vi "TekAFG3102_2.vi"() -> ()   [LabVIEW 2015]
uses:
  Shared program Control/loop state machine.ctl
  NetworkStream/NetworkStreamReceiverState.ctl
  NetworkStream/NetworkStreamStateMachineVariable.ctl
  NetworkStream/NetworkStreamData.ctl
  Shared program Control/MasterStatus.ctl
  <vilib>/dex/Stream Element Allocation Mode.ctl
  ICcamera/MyToolsFunction.lvlib
  Tek shared libraries/ArbitraryFunctions.lvlib
  NetworkStream/NetworkStream.lvlib
  Shared program Control/MySharedVariables.lvlib
  Tek shared libraries/SerialCommunication.lvlib
panel:
  out "error out 2":errorcluster caption="error out" {"code" format="%.0x"}
  in  "get tek parameters":bool
  out "error out":errorcluster {"code" format="%.0x"}
  in  "visa":bool
  out "Read Buffer":string
  in  "Write Buffer (\"\")":string="*IDN?"
  out "sequence number":u64
  in  "user waveform":bool
  in  "Channel 1 ON/OFF":bool
  in  "resource name":refnum<k15>
  in  "Stop Button":bool
  out "Session Hash":u64
  out "Network Stream State Indicator":T1
  in  "slot to load (update first)":i32(ring) items=["Slot 1", "Slot 2", "Slot 3", "Slot 4"]
  in  "channels":enum32{"active channel", ""}(radio)
  in  "Tab Control":T2(tab)
  in  "CM cluster":T3={"Frequency (Hz)"=80000000.0, "Amplitude (V)"=0.2, "Phase (°)"=0.0, "Offset (Volt)"=0.0, "Standard waveform (1: Sine)"=1, "output mode"=0, "Modulation Waveform (1: Sine)"=1} {"Modulation Waveform (1: Sine)" items=["Sine"=1, "Square"=2, "Triangle"=3, "Ramp Up"=4, "Ramp Down"=5, "Noise"=100, "Arbitrary User1"=200, "Arbitrary User2"=201, "Arbitrary User3"=202, "Arbitrary User4"=203, "Edit Memory"=204]; "output mode" items=["Standard Function", "Arbitrary Waveform"]; "Standard waveform (1: Sine)" items=["Sine"=1, "Square"=2, "Pulse"=1002, "Ramp"=1001, "Noise"=1003, "DC"=6, "Sin(x)/x"=1004, "Gaussian"=1005, "Lorentz"=1006, "Exponential Rise"=1007, "Exponential Decay"=1008, "Haversine"=1009]}
  in  "AM Modulation Mode Cluster":T4={"waveform (1: Sine)"=1, "depth M (%)"=50.0, "Modulation source"=0, "AM Frequency (Hz)"=10.0, "ON/OFF"=FALSE} {"Modulation source" items=["Intern", "Extern"]; "waveform (1: Sine)" items=["Sine"=1, "Square"=2, "Pulse"=1002, "Ramp"=1001, "Noise"=1003, "DC"=6, "Sin(x)/x"=1004, "Gaussian"=1005, "Lorentz"=1006, "Exponential Rise"=1007, "Exponential Decay"=1008, "Haversine"=1009]}
  in  "FM":T5={"ON/OFF"=FALSE, "source (0: Internal)"=0, "peak deviation (1000000)"=1000000.0, "modulation frequency (10000)"=10000.0, "waveform (1: Sine)"=1} {"waveform (1: Sine)" items=["Sine"=1, "Square"=2, "Pulse"=1002, "Ramp"=1001, "Noise"=1003, "DC"=6, "Sin(x)/x"=1004, "Gaussian"=1005, "Lorentz"=1006, "Exponential Rise"=1007, "Exponential Decay"=1008, "Haversine"=1009]; "source (0: Internal)" items=["Internal", "External"]}
  in  "PM Modulation Cluster":T6={"Source (0: Internal)"=0, "Peak Deviation (90)"=90.0, "ON/OFF"=FALSE, "Modulation Frequency (10000)"=32467.5, "Modulation Waveform (1: Sine)"=1} {"Modulation Waveform (1: Sine)" items=["Sine"=1, "Square"=2, "Triangle"=3, "Ramp Up"=4, "Ramp Down"=5, "Noise"=100, "Arbitrary User1"=200, "Arbitrary User2"=201, "Arbitrary User3"=202, "Arbitrary User4"=203, "Edit Memory"=204]; "Source (0: Internal)" items=["Internal", "External"]}
  in  "force trigger":bool
  out "ready":bool=TRUE
  out "loop state machine":T7=enum."load user waveform"
  # "Depth M is varied between 0% and 120% (the latter corresponding \nto a maximum amplitude of A(Vpp)). Cf p63 doc"
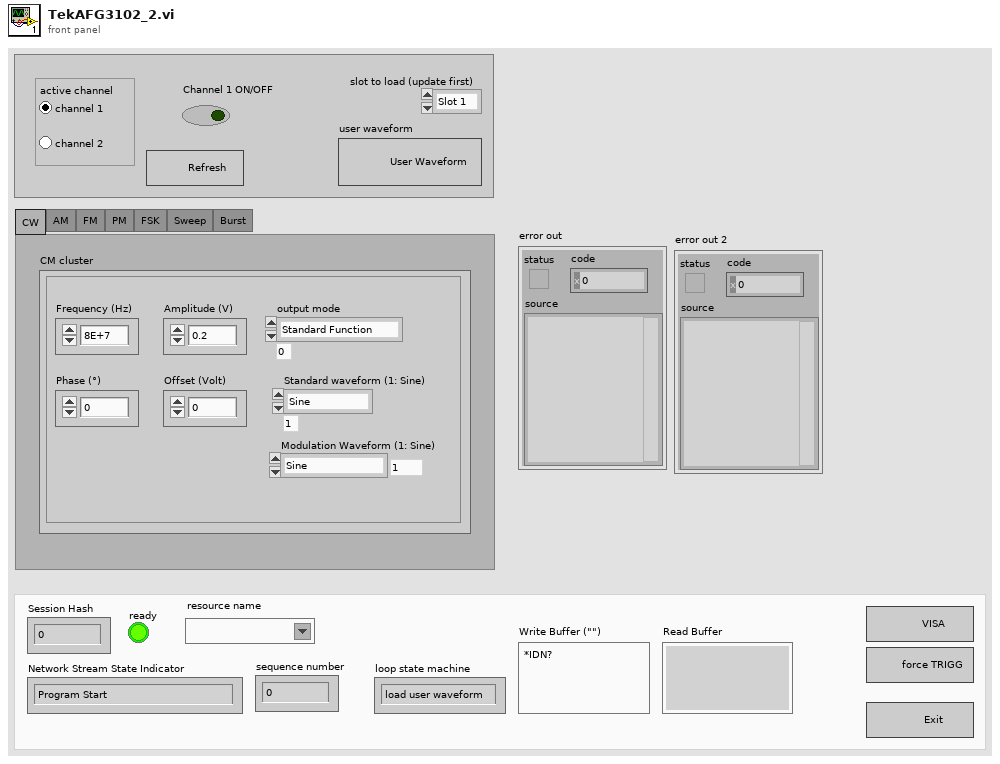
[diagram p1: front panel]
types:
  T1 = typedef "NetworkStream.lvlib/NetworkStreamReceiverState.ctl" = enum16{"Program Start", "Waiting for connection", "Connected", "Connection lost", "Exit", "Unhandled Exception"}
  T2 = enum32{"CW", "AM", "FM", "PM", "FSK", "Sweep", "Burst"}
  T3 = cluster{"Frequency (Hz)":dbl, "Amplitude (V)":dbl, "Phase (°)":dbl, "Offset (Volt)":dbl, "Standard waveform (1: Sine)":i32, "output mode":i32, "Modulation Waveform (1: Sine)":i32}
  T4 = cluster{"waveform (1: Sine)":i32, "depth M (%)":dbl, "Modulation source":u16, "AM Frequency (Hz)":dbl, "ON/OFF":bool}
  T5 = cluster{"ON/OFF":bool, "source (0: Internal)":i32, "peak deviation (1000000)":dbl, "modulation frequency (10000)":dbl, "waveform (1: Sine)":i32}
  T6 = cluster{"Source (0: Internal)":i32, "Peak Deviation (90)":dbl, "ON/OFF":bool, "Modulation Frequency (10000)":dbl, "Modulation Waveform (1: Sine)":i32}
  T7 = typedef "loop state machine.ctl" = enum16{"ready", "write on VISA", "get tek param", "load user waveform", "update channel parameters", "update status", "channel on/off", "initialize", "exit", "error"}
  T8 = typedef "MySharedVariables.lvlib/MasterStatus.ctl" = cluster{"Camera done":bool, "Tektronik done":bool, "Motors done":bool, "Gage done":bool}[]
  T9 = typedef "NetworkStream.lvlib/NetworkStreamData.ctl" = cluster{"Command/Status":string, "Data":variant, "Session Hash":u64, "Sequence Number":u64}
  T10 = typedef "NetworkStream.lvlib/NetworkStreamStateMachineVariable.ctl" = cluster{"Network Stream Reader Endpoint":refnum<k21>, "Last Received Sequence Number":u64}
  T11 = cluster{"Frequency (Hz)":dbl, "Amplitude (V)":dbl, "Phase (°)":dbl, "Offset (Volt)":dbl, "waveform (1: Sine)":i32, "output mode":i32}
  T12 = cluster{"max number of waveforms":i32, "waveform quantum":i32, "max waveform size":i32, "min waveform size":i32}
  T13 = cluster{"Camera done":bool, "Tektronik done":bool, "Motors done":bool, "Gage done":bool}
  T14 = typedef "Stream Element Allocation Mode.ctl" = u32
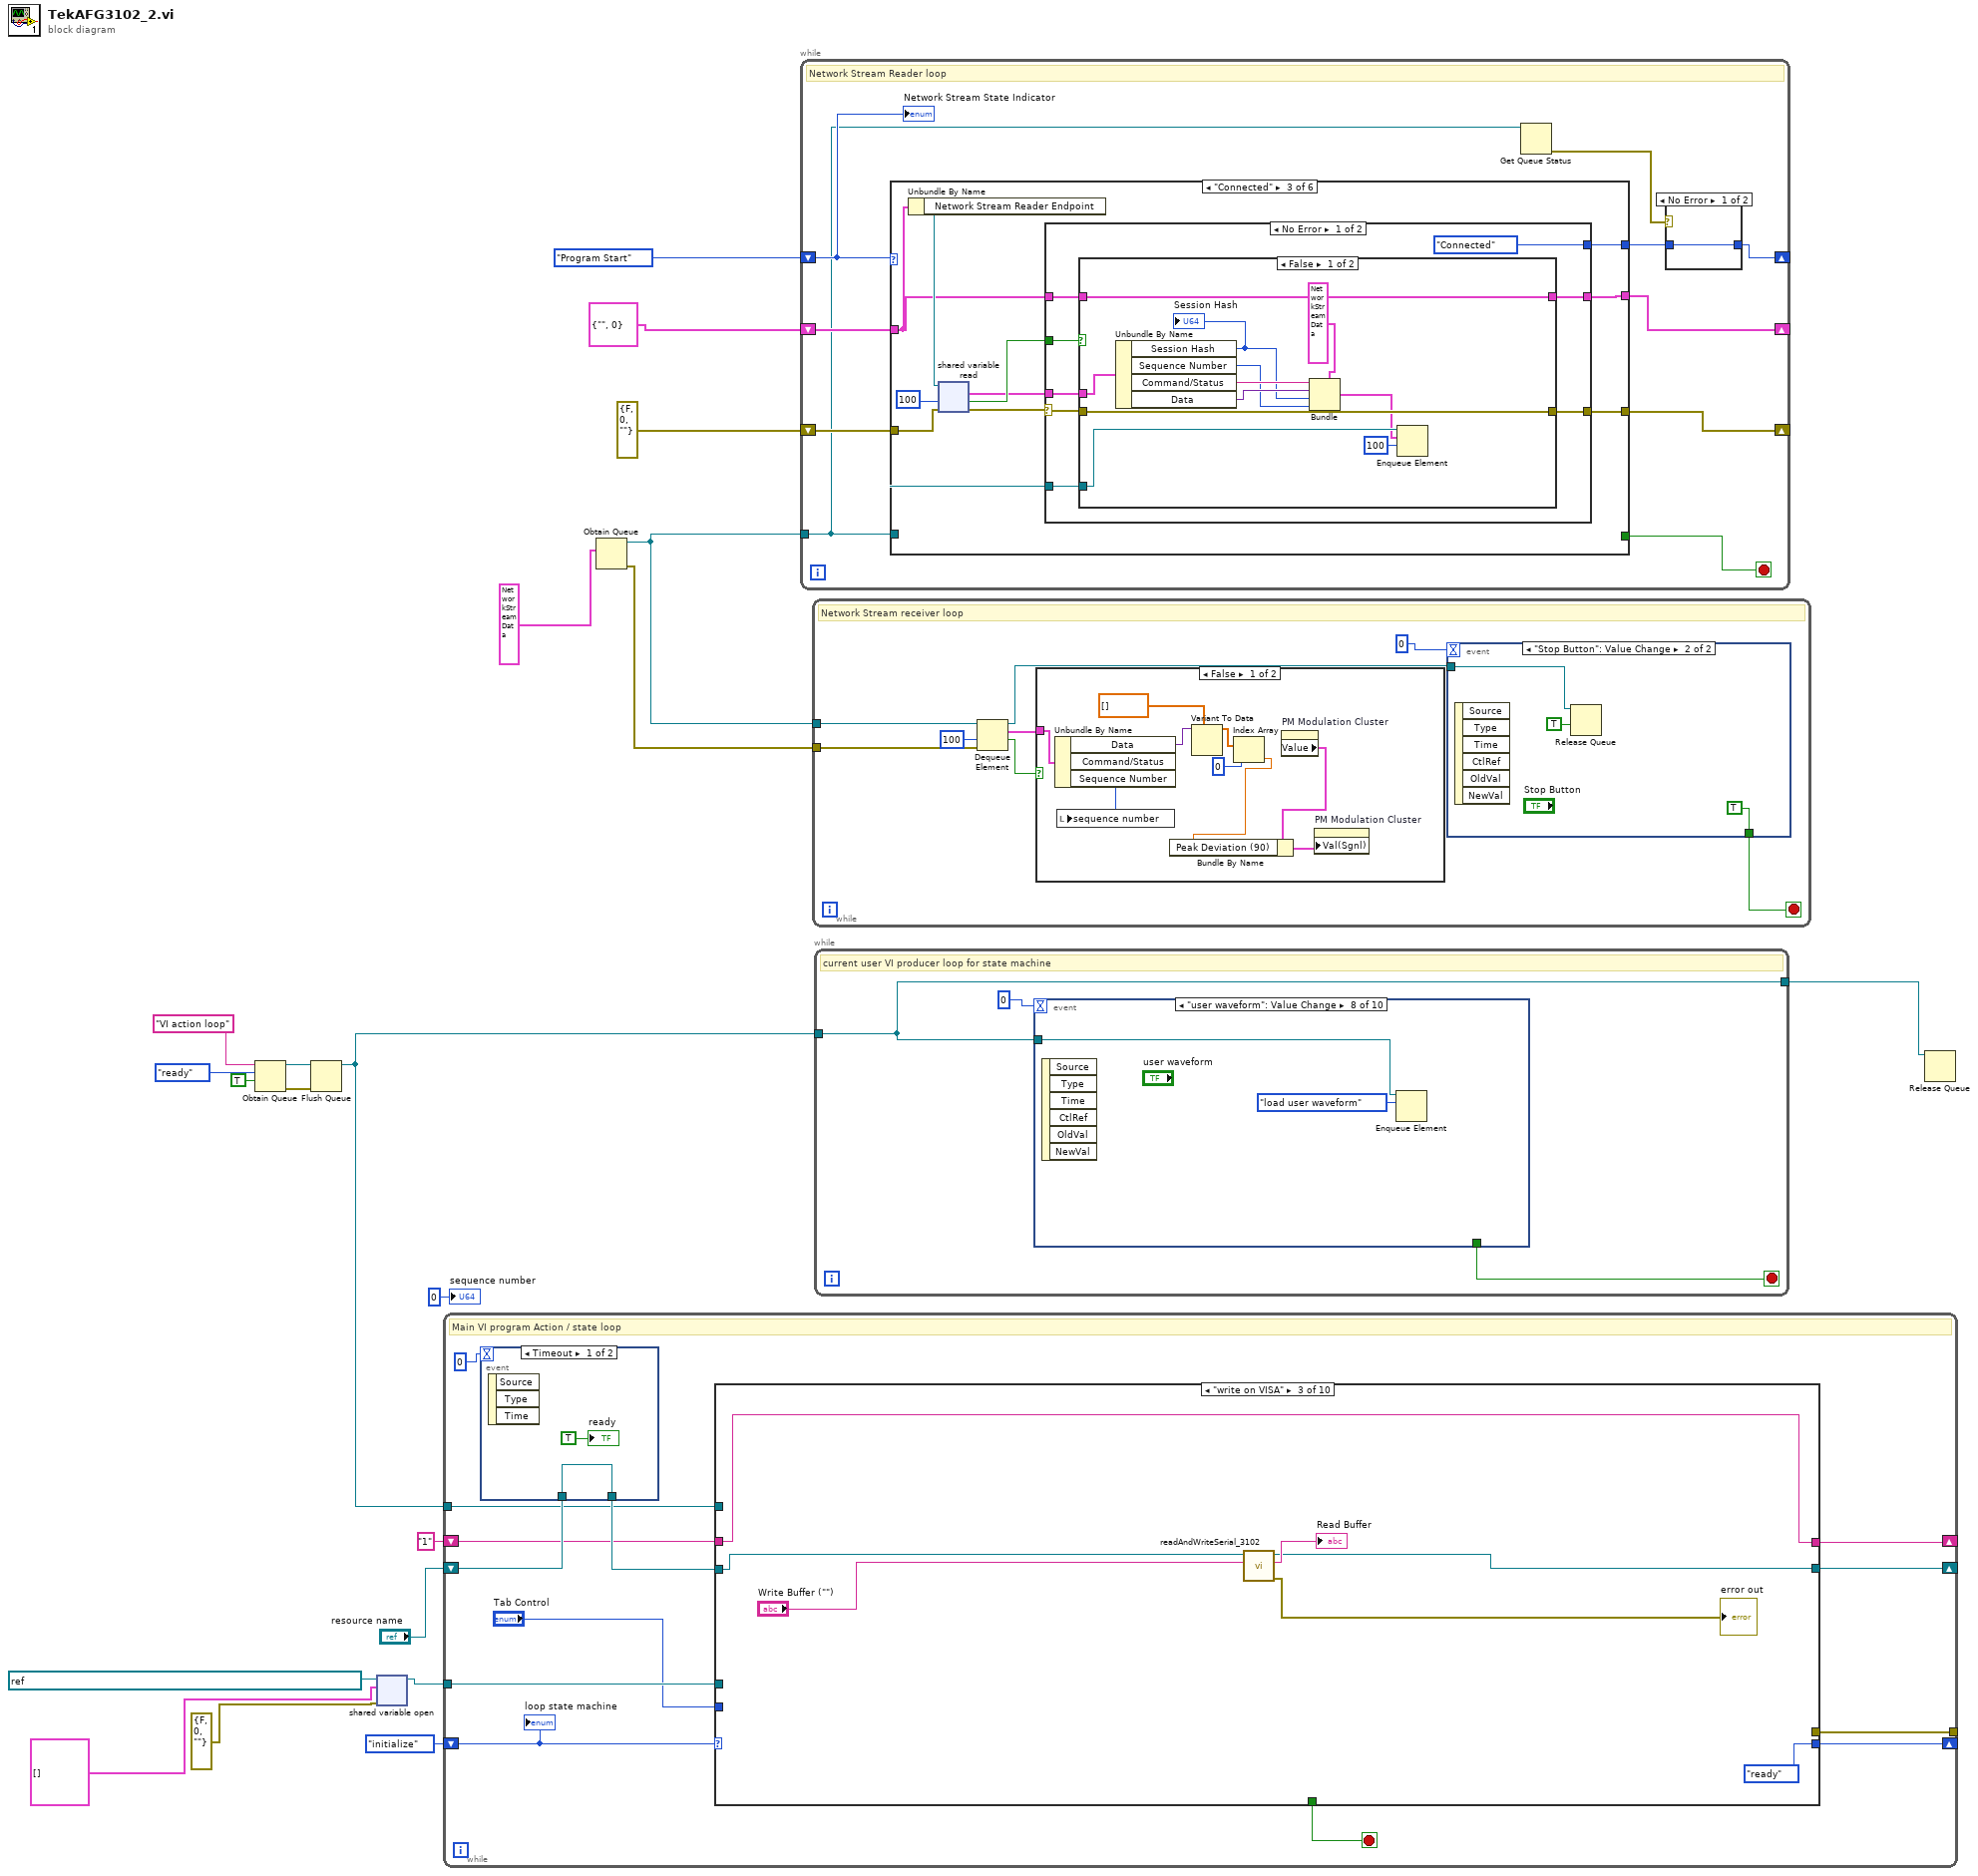
[diagram p0: block diagram]
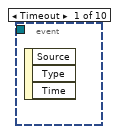
[diagram p2: hidden frame]
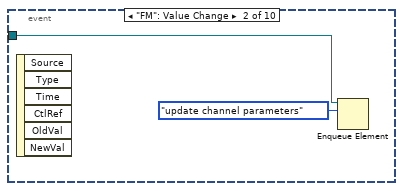
[diagram p3: hidden frame]
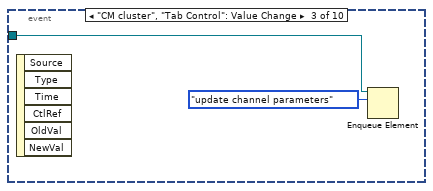
[diagram p4: hidden frame]
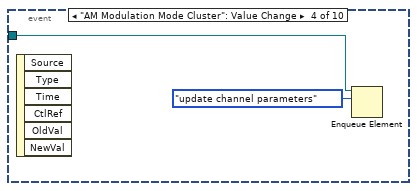
[diagram p5: hidden frame]
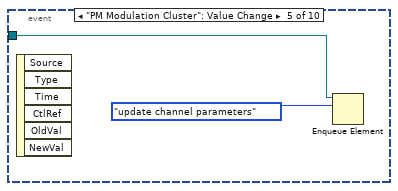
[diagram p6: hidden frame]
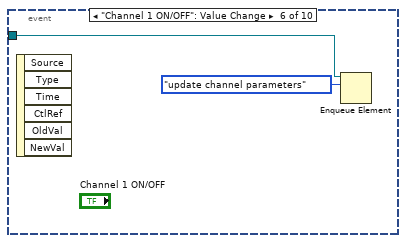
[diagram p7: hidden frame]
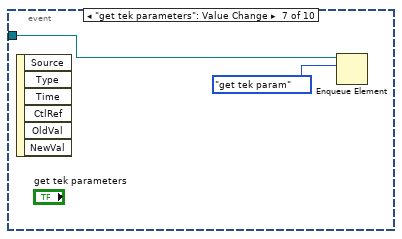
[diagram p8: hidden frame]
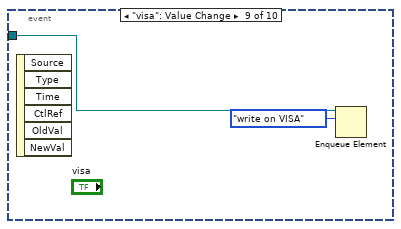
[diagram p9: hidden frame]
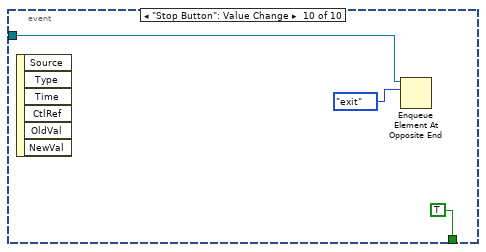
[diagram p10: hidden frame]
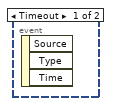
[diagram p12: hidden frame]
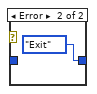
[diagram p13: hidden frame]
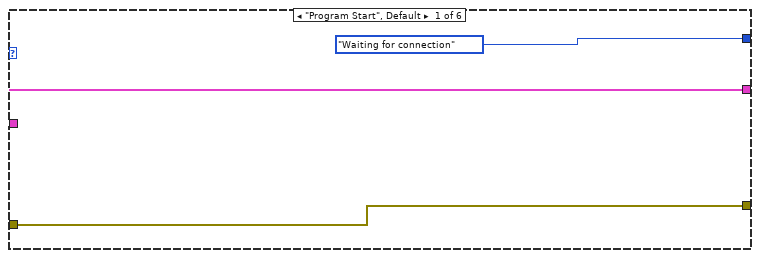
[diagram p14: hidden frame]
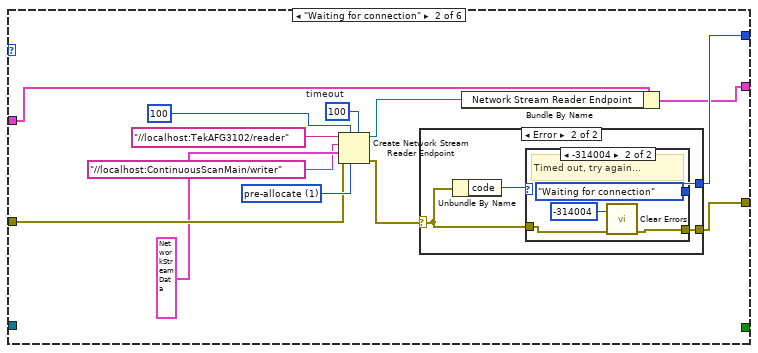
[diagram p15: hidden frame]
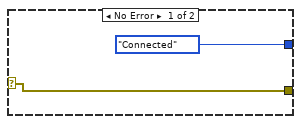
[diagram p16: hidden frame]
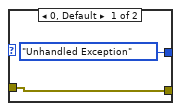
[diagram p17: hidden frame]
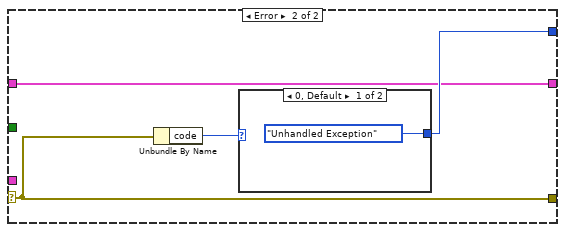
[diagram p19: hidden frame]
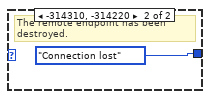
[diagram p20: hidden frame]
diagram:
  n1 = Obtain Queue(name (unnamed)="VI action loop", element data type=loop_state_machine."ready" ("loop state machine"), create if not found? (T)=TRUE) -> (queue out=w8:refnum<queue>, error out=w6:errorcluster)  [unwired: 2 in, 1 out]
  n2 = Flush Queue(queue=w8, error in (no error)=w6) -> (queue out=w7:refnum<queue>)  [unwired: 2 out]
  n3 = shared-variable-open(refnum<k21> "ni.var.psp://localhost/MySharedVariables/MasterStatusShared" ("shared variable refnum in"), errorcluster {"status"=FALSE, "code"=0, "source"=""} ("error in (no error)"), T8 [] ("MasterStatusShared")) -> (w3:refnum<k21>)  [unwired: 1 in, 1 out]
  n4 = while {
    tunnel: [w33] -> _
    shift-right: [w32] -> _
    shift-left: "resource name" -> [w27]
    shift-right: [w30] -> _
    shift-left: loop_state_machine."initialize" ("loop state machine") -> [w31]
    shift-right: [w28] -> _
    shift-left: "1" -> [w25]
    tunnel: w7 -> [w24]
    tunnel: w3 -> [w23]
    stop <- w34 stop-if-true
    # "Main VI program Action / state loop"
    n5 = event shown="[0] Timeout" {
      selector: _ -> [_ _]
      dyn-events: _ -> [_ _]
      timeout: 0 -> [_ _]
      tunnel: w27 -> [w35 w37]
      tunnel: [w35 w37] -> w26
      event Timeout {
        n6 = event-data() -> ()  [unwired: 1 in, 3 out]
        "ready" <- TRUE
      }
      event "force trigger": Value Change {
        n7 = event-data() -> ()  [unwired: 1 in, 3 out]
      }
    }
    n8 = case shown="\"write on VISA\"" w31 {
      tunnel: [_ _ _ TRUE _ _ _ _ _ _] -> w34
      tunnel: [w43 w55 _ w69 errorcluster {"status"=FALSE, "code"=0, "source"=""} ("error out") errorcluster {"status"=FALSE, "code"=0, "source"=""} ("error out") w89 w154 w170 errorcluster {"status"=FALSE, "code"=0, "source"=""} ("error out")] -> w33
      tunnel: [w40 w57 w60 w70 w81 w86 w92 w153 w173 w179] -> w32
      tunnel: [w44 loop_state_machine."ready" ("loop state machine") loop_state_machine."ready" ("loop state machine") loop_state_machine."exit" ("loop state machine") w78 loop_state_machine."exit" ("loop state machine") loop_state_machine."update status" ("loop state machine") loop_state_machine."ready" ("loop state machine") loop_state_machine."ready" ("loop state machine") loop_state_machine."ready" ("loop state machine")] -> w30
      tunnel: w26 -> [w42 w58 w63 w70 w81 w86 w93 w164 w174 w179]
      tunnel: [w39 w56 w64 w67 w80 w87 w91 w152 w172 w180] -> w28
      tunnel: w25 -> [w39 w56 w64 w67 w80 w87 _ w152 w172 w180]
      tunnel: w24 -> [_ _ _ _ w74 _ _ _ _ _]
      tunnel: w23 -> [_ _ _ w66 _ _ _ _ _ w176]
      tunnel: "Tab Control" -> [_ _ _ _ _ _ w88 _ _ _]
      frame "initialize", Default {
        n9 = call <instrlib>:"tkafg3k Initialize.vi"("error in (no error)"=errorcluster {"status"=FALSE, "code"=0, "source"=""}, "reset device (Yes)"=FALSE, "resource name"=w42) -> ("error out"=w47:errorcluster, "instrument handle out"=w45:refnum<k15>)  [unwired: 7 in]
        n10 = call <instrlib>:"tkafg3k Clear Arbitrary Waveform.vi"("error in (no error)"=w47, "waveform handle"=-1, "instrument handle"=w45) -> ("error out"=w43:errorcluster, "instrument handle out"=w41:refnum<k15>)  [unwired: 7 in]
        n11 = case shown="No Error" w43 {
          tunnel: [loop_state_machine."ready" ("loop state machine") loop_state_machine."exit" ("loop state machine")] -> w44
          tunnel: w41 -> [w49 w51]
          tunnel: [w49 w51] -> w40
          frame No Error {
          }
          frame Error {
          }
        }
      }
      frame "get tek param" {
        n12 = control-ref of="Tab Control"() -> (w53:refnum<vi>)
        n13 = call "GetModeSatus.vi"("Tab Control"=w53, "instrument handle"=w58) -> ("error out"=w55:errorcluster, "instrument handle out"=w57:refnum<k15>)  [unwired: 6 in, 2 out]
        "error out 2" <- w55
      }
      frame "write on VISA" {
        n14 = call "readAndWriteSerial_3102.vi"("Write Buffer (\"\")"="Write Buffer (\"\")", "instrument handle"=w63) -> ("error out"=→"error out":errorcluster, "Read Buffer"=→"Read Buffer":string, "instrument handle out"=w60:refnum<k15>)  [unwired: 6 in, 1 out]
      }
      frame "exit" {
        n15 = Close Variable Connection(11:w66) -> ()  [unwired: 1 in, 1 out]
        n16 = call <instrlib>:"tkafg3k Close.vi"("instrument handle"=w70) -> ("error out"=w71:errorcluster)  [unwired: 10 in]
        n17 = call <vilib>:"Simple Error Handler.vi"("error in (no error)"=w71) -> ("error out"=w69:errorcluster)  [unwired: 1 in, 7 out]
      }
      frame "ready" {
        n18 = Get Queue Status(queue=w74) -> (queue out=w73:refnum<queue>)  [unwired: 2 in, 7 out]
        n19 = Dequeue Element(queue=w73, timeout in ms (-1)=200) -> (element=w76:T7, error out=w77:errorcluster)  [unwired: 1 in, 2 out]
        n20 = case shown="No Error" w77 {
          tunnel: [w82 loop_state_machine."exit" ("loop state machine")] -> w78
          tunnel: w76 -> [w82 _]
          frame No Error {
          }
          frame Error {
          }
        }
      }
      frame "error" {
      }
      frame "update channel parameters" {
        n21 = case shown="\"active channel\", Default" "channels" {
          tunnel: ["1" "2"] -> w94
          frame "active channel", Default {
            n22 = property on="ready" class="Bool (strict)"("Value"=FALSE ("ready")) -> ()  [unwired: 2 in, 2 out]
          }
          frame "" {
            n23 = property on="ready" class="Bool (strict)"("Value"=FALSE ("ready")) -> ()  [unwired: 2 in, 2 out]
          }
        }
        n24 = case shown="\"PM\"" w88 {
          tunnel: w94 -> [w96 w105 w113 w118 w126 w131 w136]
          tunnel: w93 -> [w103 w112 w116 w125 w130 w135 w142]
          tunnel: [w99 w107 w115 w120 w129 w133 w138] -> w92
          tunnel: [w101 w109 w114 w122 w128 w132 w140] -> w89
          tunnel: [w96 w105 w113 w118 w126 w131 w136] -> w91
          frame "CW", Default {
            w104 = 0 items=["Continuous"=0, "Modulation"=1001, "Sweep"=1002, "Burst"=1] ("operation mode (0: Continuous)")
            n25 = call <instrlib>:"tkafg3k Configure Operation Mode.vi"("operation mode (0: Continuous)"=w104, "channel name (\"1\")"=w96, "instrument handle"=w103) -> ("error out"=w102:errorcluster, "instrument handle out"=w100:refnum<k15>)  [unwired: 7 in]
            n26 = call "Update_CW.vi"("channel name (\"1\")"=w96, "error in (no error)"=w102, "CM cluster"="CM cluster", "resource name"=w100) -> ("error out"=w101:errorcluster, "output cluster"=w97:T11, "instrument handle out"=w99:refnum<k15>)  [unwired: 5 in]
            n27 = Unbundle By Name(w97) -> ()  [unwired: 1 out]
          }
          frame "FM" {
            w111 = 1001 items=["Continuous"=0, "Modulation"=1001, "Sweep"=1002, "Burst"=1] ("operation mode (0: Continuous)")
            n28 = call <instrlib>:"tkafg3k Configure Operation Mode.vi"("operation mode (0: Continuous)"=w111, "channel name (\"1\")"=w105, "instrument handle"=w112) -> ("error out"=w110:errorcluster, "instrument handle out"=w108:refnum<k15>)  [unwired: 7 in]
            n29 = call "Update_FM.vi"("error in (no error)"=w110, "channel name (\"1\")"=w105, "FM"="FM", "resource name"=w108) -> ("error out"=w109:errorcluster, "instrument handle out"=w107:refnum<k15>)  [unwired: 5 in, 1 out]
          }
          frame "FSK" {
            w117 = 1001 items=["Continuous"=0, "Modulation"=1001, "Sweep"=1002, "Burst"=1] ("operation mode (0: Continuous)")
            n30 = call <instrlib>:"tkafg3k Configure Operation Mode.vi"("operation mode (0: Continuous)"=w117, "channel name (\"1\")"=w113, "instrument handle"=w116) -> ("error out"=w114:errorcluster, "instrument handle out"=w115:refnum<k15>)  [unwired: 7 in]
          }
          frame "PM" {
            w124 = 1001 items=["Continuous"=0, "Modulation"=1001, "Sweep"=1002, "Burst"=1] ("operation mode (0: Continuous)")
            n31 = call <instrlib>:"tkafg3k Configure Operation Mode.vi"("operation mode (0: Continuous)"=w124, "channel name (\"1\")"=w118, "instrument handle"=w125) -> ("error out"=w123:errorcluster, "instrument handle out"=w121:refnum<k15>)  [unwired: 7 in]
            n32 = call "Update_PM.vi"("PM Modulation Cluster"="PM Modulation Cluster", "error in (no error)"=w123, "channel name (\"1\")"=w118, "resource name"=w121) -> ("error out"=w122:errorcluster, "instrument handle out"=w120:refnum<k15>)  [unwired: 5 in, 1 out]
          }
          frame "Sweep" {
            w127 = 1002 items=["Continuous"=0, "Modulation"=1001, "Sweep"=1002, "Burst"=1] ("operation mode (0: Continuous)")
            n33 = call <instrlib>:"tkafg3k Configure Operation Mode.vi"("operation mode (0: Continuous)"=w127, "channel name (\"1\")"=w126, "instrument handle"=w130) -> ("error out"=w128:errorcluster, "instrument handle out"=w129:refnum<k15>)  [unwired: 7 in]
          }
          frame "Burst" {
            w134 = 1 items=["Continuous"=0, "Modulation"=1001, "Sweep"=1002, "Burst"=1] ("operation mode (0: Continuous)")
            n34 = call <instrlib>:"tkafg3k Configure Operation Mode.vi"("operation mode (0: Continuous)"=w134, "channel name (\"1\")"=w131, "instrument handle"=w135) -> ("error out"=w132:errorcluster, "instrument handle out"=w133:refnum<k15>)  [unwired: 7 in]
          }
          frame "AM" {
            w143 = 1001 items=["Continuous"=0, "Modulation"=1001, "Sweep"=1002, "Burst"=1] ("operation mode (0: Continuous)")
            n35 = call <instrlib>:"tkafg3k Configure Operation Mode.vi"("operation mode (0: Continuous)"=w143, "channel name (\"1\")"=w136, "instrument handle"=w142) -> ("error out"=w141:errorcluster, "instrument handle out"=w139:refnum<k15>)  [unwired: 7 in]
            n36 = call "Update_AM.vi"("AM Modulation Mode Cluster"="AM Modulation Mode Cluster", "error in (no error)"=w141, "channel name (\"1\")"=w136, "resource name"=w139) -> ("error out"=w140:errorcluster, "instrument handle out"=w138:refnum<k15>)  [unwired: 5 in, 1 out]
          }
        }
      }
      frame "load user waveform" {
        n37 = property on="ready" class="Bool (strict)"("Value"=FALSE ("ready")) -> (error out=w150:errorcluster)  [unwired: 2 in, 1 out]
        n38 = call <instrlib>:"tkafg3k Query Arb Waveform Capabilities.vi"("error in (no error)"=w150, "instrument handle"=w164) -> ("error out"=w157:errorcluster, "waveform quantum"=w168:i32, "max number of waveforms"=w167:i32, "instrument handle out"=w158:refnum<k15>, "max waveform size"=w163:i32, "min waveform size"=w162:i32)  [unwired: 4 in]
        n39 = property on="PM Modulation Cluster" class="Clust (strict)"() -> ("Value"=w149:T6)  [unwired: 2 in, 2 out]
        n40 = Bundle("max number of waveforms"=w167, "waveform quantum"=w168, "max waveform size"=w163, "min waveform size"=w162) -> (w161:T12)  [unwired: 1 in]
        n41 = Unbundle By Name(w149) -> ("Modulation Frequency (10000)"=w148:dbl)
        n42 = call "LoadWaveForm.vi"("modulation frequency (Hz)"=w148, "Npoint"=1000.0 ("arbitrary frequency (Npoints)"), "arbitrary parameters"=w161) -> ("waveform"=w151:dbl[])  [unwired: 8 in]
        n43 = Array Size(array=w151) -> (size(s)=w156:i32)
        n44 = call <instrlib>:"tkafg3k Create Arbitrary Waveform by Slot.vi"("overwrite (False)"=TRUE, "slot (0: Slot 1)"="slot to load (update first)", "error in (no error)"=w157, "waveform data array"=w151, "waveform size (1000)"=w156, "instrument handle"=w158) -> ("error out"=w154:errorcluster, "instrument handle out"=w153:refnum<k15>)  [unwired: 4 out]
      }
      frame "channel on/off" {
        n45 = property on="Channel 1 ON/OFF" class="Bool (strict)"() -> ("Value"=w171:bool)  [unwired: 2 in, 2 out]
        n46 = call <instrlib>:"tkafg3k Configure Output Enabled.vi"("channel enabled (True)"=w171, "channel name (\"1\")"=w172, "instrument handle"=w174) -> ("error out"=w170:errorcluster, "instrument handle out"=w173:refnum<k15>)  [unwired: 7 in]
      }
      frame "update status" {
        n47 = property on="Network Stream State Indicator" class="Enum (strict)"() -> ("Value"=w175:T1)  [unwired: 2 in, 2 out]
        n48 = case shown="\"Connected\"" w175 {
          tunnel: w176 -> [_ w186]
          frame "Program Start", Default {
          }
          frame "Connected" {
            n49 = local read "sequence number"() -> (w184:u64)
            n50 = shared-variable-read(w186) -> (w188:refnum<k21>, w185:T8)  [unwired: 1 in, 2 out]
            n51 = Index Array(array=w185, index=w184) -> (element=w183:T13)
            n52 = Bundle By Name(cluster=w183, "Tektronik done"=TRUE) -> (w182:T13)
            n53 = Replace Array Subset(array=w185, new element=w182, index=w184) -> (w187:T8)
            n54 = shared-variable-write(w188, w187) -> ()  [unwired: 1 in, 2 out]
          }
        }
      }
    }
    "loop state machine" <- w31
  }
  n55 = Obtain Queue(element data type=T9 {"Command/Status"="", "Data"=variant, "Session Hash"=0, "Sequence Number"=0} ("NetworkStreamCluster")) -> (queue out=w17:refnum<queue>, error out=w18:errorcluster)  [unwired: 4 in, 1 out]
  n56 = while {
    shift-right: [w196] -> _
    shift-left: T10 {"Network Stream Reader Endpoint"="", "Last Received Sequence Number"=0} ("StateMachineVariable") -> [w198]
    shift-right: [w191] -> _
    shift-left: NetworkStreamReceiverState."Program Start" -> [w197]
    shift-right: [w195] -> _
    shift-left: errorcluster {"status"=FALSE, "code"=0, "source"=""} ("error in (no error)") -> [w193]
    tunnel: w17 -> [w189]
    stop <- w194 stop-if-true
    # "Network Stream Reader loop"
    n57 = case shown="\"Connected\"" w197 {
      tunnel: [NetworkStreamReceiverState."Waiting for connection" w212 w234 NetworkStreamReceiverState."Waiting for connection" NetworkStreamReceiverState."Exit" NetworkStreamReceiverState."Exit"] -> w192
      tunnel: [w202 w211 w235 w271 w284 w292] -> w195
      tunnel: [w201 w210 w232 w267 w277 w289] -> w196
      tunnel: [_ _ _ _ TRUE _] -> w194
      tunnel: w198 -> [w201 w208 w231 w268 w278 w289]
      tunnel: w193 -> [w202 w207 w230 w270 w279 w290]
      tunnel: w189 -> [_ _ w229 _ _ _]
      frame "Program Start", Default {
      }
      frame "Waiting for connection" {
        w209 = T14 1 items=["allocate as needed", "pre-allocate"] ("element allocation mode")
        w216 = 100  # timeout
        n58 = Create Network Stream Reader Endpoint(5:w216, 6:w209, 7:100 ("reader buffer size"), 8:w207, 9:T9 {"Command/Status"="", "Data"=variant, "Session Hash"=0, "Sequence Number"=0} ("NetworkStreamCluster"), 10:"//localhost:ContinuousScanMain/writer" ("writer url"), 11:"//localhost:TekAFG3102/reader" ("reader name")) -> (0:w213:errorcluster, 3:w205:refnum<k21>)
        n59 = case shown="Error" w213 {
          selector: w213 -> [w217 w220]
          tunnel: [NetworkStreamReceiverState."Connected" w222] -> w212
          tunnel: [w217 w219] -> w211
          frame No Error {
          }
          frame Error {
            n60 = Unbundle By Name(w220) -> ("code"=w221:i32)
            n61 = case shown="-314004" w221 {
              tunnel: [NetworkStreamReceiverState."Unhandled Exception" NetworkStreamReceiverState."Waiting for connection"] -> w222
              tunnel: w220 -> [w223 w226]
              tunnel: [w223 w225] -> w219
              frame 0, Default {
              }
              frame -314004 {
                # "Timed out, try again..."
                n62 = call <vilib>:"Clear Errors.vi"("error in (no error)"=w226, "specific error code to clear (0: all)"=-314004) -> ("error out"=w225:errorcluster)  [unwired: 4 in, 1 out]
              }
            }
          }
        }
        n63 = Bundle By Name(cluster=w208, "Network Stream Reader Endpoint"=w205) -> (w210:T10)
      }
      frame "Connected" {
        n64 = Unbundle By Name(w231) -> ("Network Stream Reader Endpoint"=w233:refnum<k21>)
        n65 = shared-variable-read(w233, w230, 100 ("timeout ms (-1)")) -> (w236:errorcluster, w238:bool, w237:T9)  [unwired: 1 out]
        n66 = case shown="No Error" w236 {
          selector: w236 -> [w245 w264]
          tunnel: w238 -> [w247 _]
          tunnel: w237 -> [w246 _]
          tunnel: [w244 w264] -> w235
          tunnel: [NetworkStreamReceiverState."Connected" w262] -> w234
          tunnel: [w242 w261] -> w232
          tunnel: w231 -> [w241 w261]
          tunnel: w229 -> [w240 _]
          frame No Error {
            n67 = case shown="False" w247 {
              tunnel: [w254 w260] -> w244
              tunnel: w245 -> [w254 w260]
              tunnel: w246 -> [w258 _]
              tunnel: [w255 w259] -> w242
              tunnel: w241 -> [w255 w259]
              tunnel: w240 -> [w253 _]
              frame False {
                n68 = Unbundle By Name(w258) -> ("Session Hash"=w250:u64, "Sequence Number"=w249:u64, "Command/Status"=w257:string, "Data"=w256:variant)
                "Session Hash" <- w250
                n69 = Bundle(cluster=T9 {"Command/Status"="", "Data"=variant, "Session Hash"=0, "Sequence Number"=0} ("NetworkStreamCluster"), "Command/Status"=w257, "Data"=w256, "Session Hash"=w250, "Sequence Number"=w249) -> (w252:T9)
                n70 = Enqueue Element(queue=w253, element=w252, timeout in ms (-1)=100) -> ()  [unwired: 1 in, 3 out]
              }
              frame True {
              }
            }
          }
          frame Error {
            n71 = Unbundle By Name(w264) -> ("code"=w263:i32)
            n72 = case shown="0, Default" w263 {
              tunnel: [NetworkStreamReceiverState."Unhandled Exception" NetworkStreamReceiverState."Connection lost"] -> w262
              frame 0, Default {
              }
              frame -314310, -314220 {
                # "The remote endpoint has been destroyed."
              }
            }
          }
        }
      }
      frame "Connection lost" {
        w274 = refnum<k21> refnum  # reader endpoint
        n73 = Unbundle By Name(w268) -> ("Network Stream Reader Endpoint"=w269:refnum<k21>)
        n74 = Destroy Stream Endpoint(8:w270, 11:w269) -> (0:w273:errorcluster)
        n75 = Bundle By Name(cluster=w268, "Network Stream Reader Endpoint"=w274) -> (w267:T10)
        n76 = call <vilib>:"Clear Errors.vi"("error in (no error)"=w273, "specific error code to clear (0: all)"=0) -> ("error out"=w271:errorcluster)  [unwired: 4 in, 1 out]
      }
      frame "Exit" {
        w280 = refnum<k21> refnum  # reader endpoint
        n77 = Unbundle By Name(w278) -> ("Network Stream Reader Endpoint"=w276:refnum<k21>)
        n78 = Not Equal?(x=w280, y=w276) -> (x != y?=w282:bool)
        n79 = case shown="True" w282 {
          tunnel: [w285 w288] -> w284
          tunnel: w279 -> [w285 w287]
          tunnel: w276 -> [_ w286]
          frame False {
          }
          frame True {
            n80 = Destroy Stream Endpoint(8:w287, 11:w286) -> (0:w288:errorcluster)
          }
        }
        n81 = Bundle By Name(cluster=w278, "Network Stream Reader Endpoint"=w280) -> (w277:T10)
      }
      frame "Unhandled Exception" {
        n82 = call <vilib>:"General Error Handler.vi"("error in (no error)"=w290) -> ("error out"=w292:errorcluster)  [unwired: 10 in, 4 out]
      }
    }
    n83 = Get Queue Status(queue=w189) -> (error out=w190:errorcluster)  [unwired: 2 in, 7 out]
    n84 = case shown="No Error" w190 {
      tunnel: w192 -> [w199 _]
      tunnel: [w199 NetworkStreamReceiverState."Exit"] -> w191
      frame No Error {
      }
      frame Error {
      }
    }
    "Network Stream State Indicator" <- w197
  }
  n85 = while {
    tunnel: w18 -> [w294]
    tunnel: w17 -> [w295]
    stop <- w300 stop-if-true
    # "Network Stream receiver loop"
    n86 = Dequeue Element(queue=w295, timeout in ms (-1)=100, error in (no error)=w294) -> (queue out=w296:refnum<queue>, element=w298:T9, timed out?=w293:bool)  [unwired: 1 out]
    n87 = case shown="False" w293 {
      tunnel: w298 -> [w309 _]
      frame False {
        n88 = Unbundle By Name(w309) -> ("Data"=w306:variant, "Sequence Number"=w308:u64)  [unwired: 1 out]
        n89 = local write "sequence number"(w308) -> ()
        n90 = Variant To Data(type=dbl[] [] ("subarray 2"), Variant=w306) -> (data=w305:dbl[])  [unwired: 1 in, 1 out]
        n91 = Index Array(array=w305, index=0) -> (element=w303:dbl)
        n92 = property on="PM Modulation Cluster" class="Clust (strict)"() -> ("Value"=w302:T6)  [unwired: 2 in, 2 out]
        n93 = Bundle By Name(cluster=w302, "Peak Deviation (90)"=w303) -> (w301:T6)
        n94 = property on="PM Modulation Cluster" class="Clust (strict)"("Val(Sgnl)"=w301) -> ()  [unwired: 2 in, 2 out]
      }
      frame True {
      }
    }
    n95 = event shown="[1] \"Stop Button\": Value Change" {
      selector: _ -> [_ _]
      dyn-events: _ -> [_ _]
      timeout: 0 -> [_ _]
      tunnel: [_ TRUE] -> w300
      tunnel: w296 -> [_ w311]
      event Timeout {
        n96 = event-data() -> ()  [unwired: 1 in, 3 out]
      }
      event "Stop Button": Value Change {
        n97 = event-data() -> ()  [unwired: 1 in, 6 out]
        n98 = Release Queue(queue=w311, force destroy? (F)=TRUE) -> ()  [unwired: 1 in, 3 out]
      }
    }
  }
  n99 = while {
    tunnel: w7 -> [w314]
    tunnel: [w314] -> w10
    stop <- w313 stop-if-true
    # "current user VI producer loop for state machine"
    n100 = event shown="[7] \"user waveform\": Value Change" {
      selector: _ -> [_ _ _ _ _ _ _ _ _ _]
      dyn-events: _ -> [_ _ _ _ _ _ _ _ _ _]
      timeout: 0 -> [_ _ _ _ _ _ _ _ _ _]
      tunnel: w314 -> [_ w316 w318 w320 w322 w324 w327 w328 w331 w334]
      tunnel: [_ _ _ _ _ _ _ _ _ TRUE] -> w313
      event Timeout {
        n101 = event-data() -> ()  [unwired: 1 in, 3 out]
      }
      event "FM": Value Change {
        n102 = event-data() -> ()  [unwired: 1 in, 6 out]
        n103 = Enqueue Element(queue=w316, element=loop_state_machine."update channel parameters") -> ()  [unwired: 2 in, 3 out]
      }
      event "CM cluster", "Tab Control": Value Change {
        n104 = event-data() -> ()  [unwired: 1 in, 6 out]
        n105 = Enqueue Element(queue=w318, element=loop_state_machine."update channel parameters") -> ()  [unwired: 2 in, 3 out]
      }
      event "AM Modulation Mode Cluster": Value Change {
        n106 = event-data() -> ()  [unwired: 1 in, 6 out]
        n107 = Enqueue Element(queue=w320, element=loop_state_machine."update channel parameters") -> ()  [unwired: 2 in, 3 out]
      }
      event "PM Modulation Cluster": Value Change {
        n108 = event-data() -> ()  [unwired: 1 in, 6 out]
        n109 = Enqueue Element(queue=w322, element=loop_state_machine."update channel parameters") -> ()  [unwired: 2 in, 3 out]
      }
      event "Channel 1 ON/OFF": Value Change {
        n110 = event-data() -> ()  [unwired: 1 in, 6 out]
        n111 = Enqueue Element(queue=w324, element=loop_state_machine."update channel parameters") -> ()  [unwired: 2 in, 3 out]
      }
      event "get tek parameters": Value Change {
        n112 = event-data() -> ()  [unwired: 1 in, 6 out]
        n113 = Enqueue Element(queue=w327, element=loop_state_machine."get tek param") -> ()  [unwired: 2 in, 3 out]
      }
      event "user waveform": Value Change {
        n114 = event-data() -> ()  [unwired: 1 in, 6 out]
        n115 = Enqueue Element(queue=w328, element=loop_state_machine."load user waveform") -> ()  [unwired: 2 in, 3 out]
      }
      event "visa": Value Change {
        n116 = event-data() -> ()  [unwired: 1 in, 6 out]
        n117 = Enqueue Element(queue=w331, element=loop_state_machine."write on VISA") -> ()  [unwired: 2 in, 3 out]
      }
      event "Stop Button": Value Change {
        n118 = event-data() -> ()  [unwired: 1 in, 6 out]
        n119 = Enqueue Element At Opposite End(queue=w334, element=loop_state_machine."exit") -> ()  [unwired: 2 in, 3 out]
      }
    }
  }
  n120 = Release Queue(queue=w10) -> ()  [unwired: 2 in, 3 out]
  "sequence number" <- u64 0 ("sequence number")
